vi "Gen Dst Q by BL.vi"(8 "error in (no error)":errorcluster, 9 "target pos (backend)":dbl, 10 "Motor States in":T1, 11 "Motor Obj in":refnum<class "Motor.lvclass">) -> (0 "error out":errorcluster, 1 "Dst Q (backend)":dbl[](array[numeric]), 2 "Motor States out":T1, 3 "Motor Obj out":refnum<class "Motor.lvclass">)   [LabVIEW 2016, in "Hardware.lvlib" / "Motions.lvlib" / "Motions.lvclass"]
uses:
  <userlib>/Common Components/Hardware/Abstract System/Motions/Motions/Motions.lvclass
  <userlib>/Common Components/Hardware/Motor/Motor/Motor.lvclass
  <userlib>/Common Components/Hardware/Abstract System/Motions/Motions/Motor States.ctl
  <userlib>/Common Components/TriggerAction Q/TriggerAction Q/TriggerAction Q.lvclass
  <userlib>/Common Components/Hardware/Motor/Motor/Motor.lvclass/Motor.ctl
  <userlib>/Common Components/Hardware/Motor/Motor/Accessor/Read backlash Compensation.vi
  <userlib>/Common Components/Hardware/Motor/Motor/Accessor/Read backlash option.vi
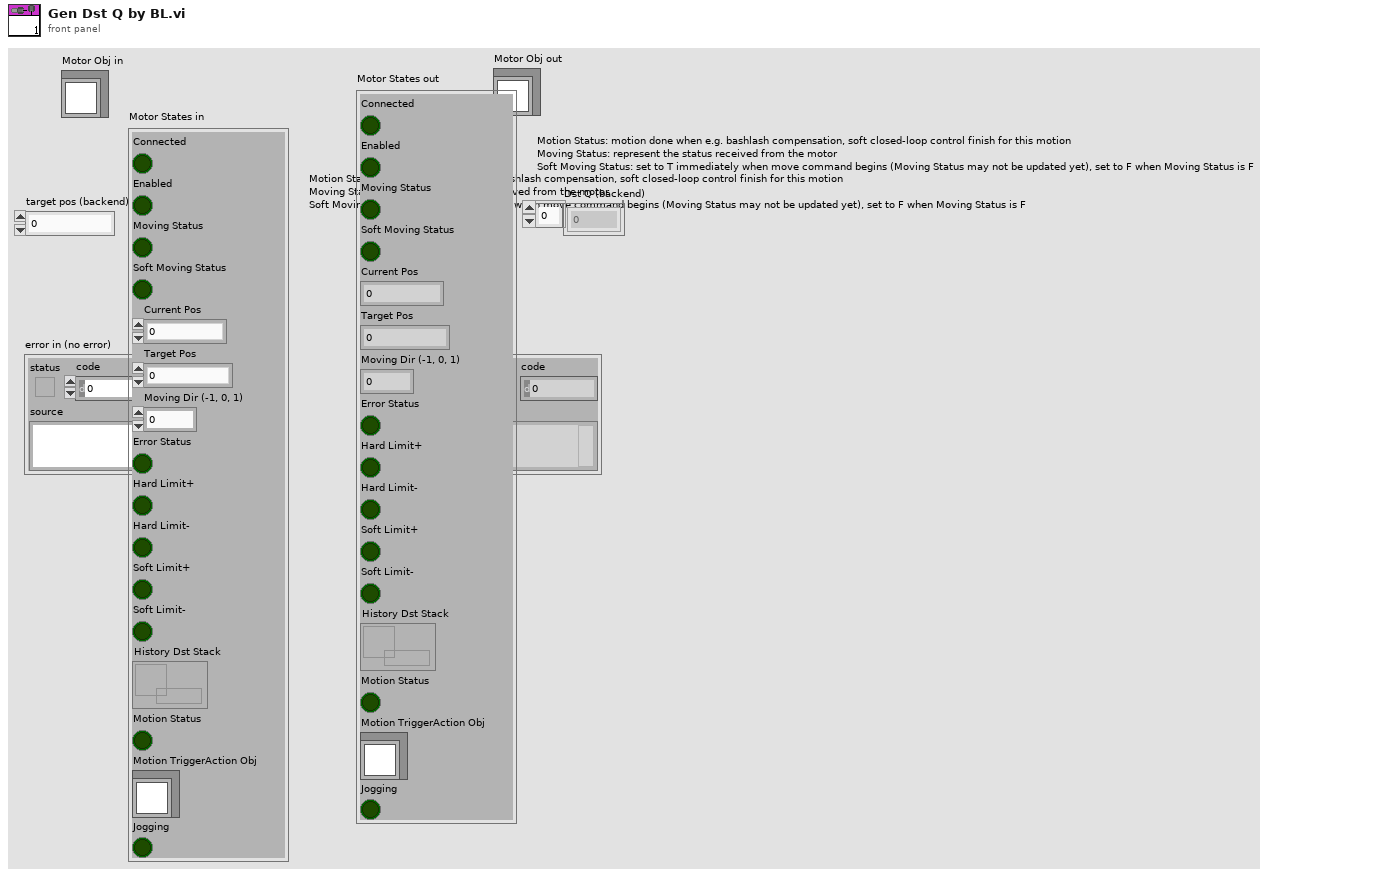
[diagram p1: front panel]
types:
  T1 = typedef "Hardware.lvlib/Motions.lvlib/Motions.lvclass/Motor States.ctl" = cluster{"Connected":bool, "Enabled":bool, "Moving Status":bool, "Soft Moving Status":bool, "Current Pos":dbl, "Target Pos":dbl, "Moving Dir (-1, 0, 1)":i32, "Error Status":bool, "Hard Limit+":bool, "Hard Limit-":bool, "Soft Limit+":bool, "Soft Limit-":bool, "History Dst Stack":refnum<queue>, "Motion Status":bool, "Motion TriggerAction Obj":refnum<class "TriggerAction Q.lvclass">, "Jogging":bool}
  T2 = enum16{"None", "arriving in + direction", "arriving in - direction"}
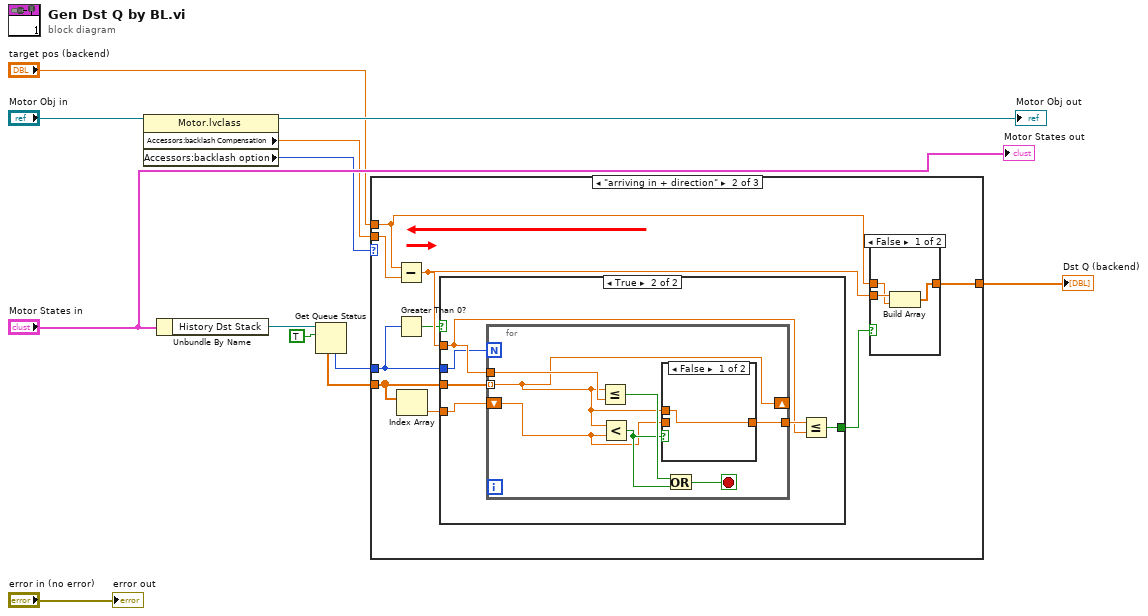
[diagram p0: block diagram]
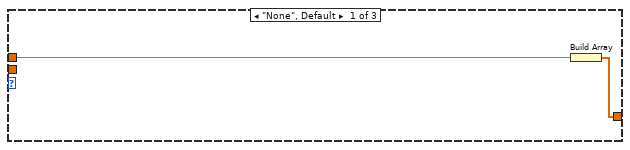
[diagram p2: hidden frame]
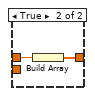
[diagram p5: hidden frame]
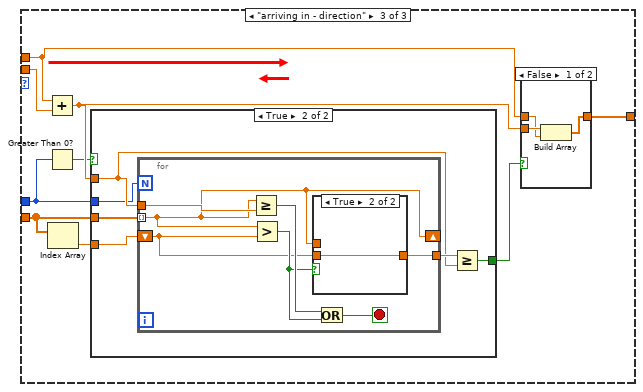
[diagram p6: hidden frame]
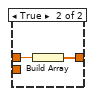
[diagram p9: hidden frame]
diagram:
  n1 = property class="Motor.lvclass"(reference="Motor Obj in") -> (reference out=→"Motor Obj out":refnum<class "Motor.lvclass">, "Accessors:backlash Compensation"=w4:dbl, "Accessors:backlash option"=w6:T2)  [unwired: 1 in, 1 out]
  n2 = Unbundle By Name("Motor States in") -> ("History Dst Stack"=w8:refnum<queue>)
  n3 = Get Queue Status(queue=w8, return elements? (F)=TRUE) -> (# elements in queue=w3:i32, elements=w2:dbl[])  [unwired: 1 in, 6 out]
  n4 = case shown="\"arriving in + direction\"" w6 {
    tunnel: w4 -> [_ w23 w52]
    tunnel: [w14 w18 w47] -> w1
    tunnel: "target pos (backend)" -> [w13 w19 w48]
    tunnel: w3 -> [_ w16 w45]
    tunnel: w2 -> [_ w21 w50]
    frame "None", Default {
      n5 = Build Array(w13) -> (w14:dbl[])
    }
    frame "arriving in + direction" {
      n6 = Subtract(x=w19, y=w23) -> (x-y=w17:dbl)
      n7 = Greater Than 0?(x=w16) -> (x > 0?=w15:bool)
      n8 = Index Array(array=w21) -> (element=w22:dbl)  [unwired: 1 in]
      n9 = case shown="True" w15 {
        tunnel: w22 -> [_ w29]
        tunnel: w21 -> [_ w28]
        tunnel: [_ w27] -> w20
        tunnel: w17 -> [_ w25]
        tunnel: w16 -> [_ w24]
        frame False {
        }
        frame True {
          n10 = for {
            N: w24 -> [_]
            tunnel: w28 -> [w31] mode=indexing
            tunnel: w25 -> [w36]
            shift-right: [w31] -> _
            shift-left: w29 -> [w32]
            tunnel: [w30] -> w26
            stop <- w34 stop-if-true
            n11 = Less Or Equal?(x=w31, y=w36) -> (x <= y?=w35:bool)
            n12 = Less?(x=w31, y=w32) -> (x < y?=w33:bool)
            n13 = case shown="False" w33 {
              tunnel: [w37 w38] -> w30
              tunnel: w32 -> [_ w38]
              tunnel: w31 -> [w37 _]
              frame False {
              }
              frame True {
              }
            }
            n14 = Or(x=w35, y=w33) -> (x .or. y?=w34:bool)
          }
          n15 = Less Or Equal?(x=w26, y=w25) -> (x <= y?=w27:bool)
        }
      }
      n16 = case shown="False" w20 {
        tunnel: w17 -> [w41 _]
        tunnel: w19 -> [w40 w43]
        tunnel: [w39 w42] -> w18
        frame False {
          n17 = Build Array(w41, w40) -> (w39:dbl[])
        }
        frame True {
          n18 = Build Array(w43) -> (w42:dbl[])
        }
      }
    }
    frame "arriving in - direction" {
      n19 = Add(x=w48, y=w52) -> (x+y=w46:dbl)
      n20 = Greater Than 0?(x=w45) -> (x > 0?=w44:bool)
      n21 = Index Array(array=w50) -> (element=w51:dbl)  [unwired: 1 in]
      n22 = case shown="True" w44 {
        tunnel: w51 -> [_ w58]
        tunnel: w50 -> [_ w57]
        tunnel: [_ w56] -> w49
        tunnel: w46 -> [_ w54]
        tunnel: w45 -> [_ w53]
        frame False {
        }
        frame True {
          n23 = for {
            N: w53 -> [_]
            tunnel: w57 -> [w60] mode=indexing
            tunnel: w54 -> [w65]
            shift-right: [w60] -> _
            shift-left: w58 -> [w61]
            tunnel: [w59] -> w55
            stop <- w63 stop-if-true
            n24 = Greater Or Equal?(x=w60, y=w65) -> (x >= y?=w64:bool)
            n25 = Greater?(x=w60, y=w61) -> (0:w62:bool)
            n26 = case shown="True" w62 {
              tunnel: [w66 w67] -> w59
              tunnel: w61 -> [_ w67]
              tunnel: w60 -> [w66 _]
              frame False {
              }
              frame True {
              }
            }
            n27 = Or(x=w64, y=w62) -> (x .or. y?=w63:bool)
          }
          n28 = Greater Or Equal?(x=w55, y=w54) -> (x >= y?=w56:bool)
        }
      }
      n29 = case shown="False" w49 {
        tunnel: w46 -> [w70 _]
        tunnel: w48 -> [w69 w72]
        tunnel: [w68 w71] -> w47
        frame False {
          n30 = Build Array(w70, w69) -> (w68:dbl[])
        }
        frame True {
          n31 = Build Array(w72) -> (w71:dbl[])
        }
      }
    }
  }
  "Dst Q (backend)" <- w1
  "error out" <- "error in (no error)"
  "Motor States out" <- "Motor States in"
